vi "Match_Proc_STD Unit.vi"(10 "Cal STD 입력":string[][](array[string]), 11 "Condition Default":string[][](array[string])) -> (1 "Cal STD 출력":string[][](array[string]), 2 "Unit":string, 3 "Condition Default out":string[][](array[string]), 4 "STD ≥ DUT?":bool, 5 "x < 0?":bool)   [LabVIEW 2020]
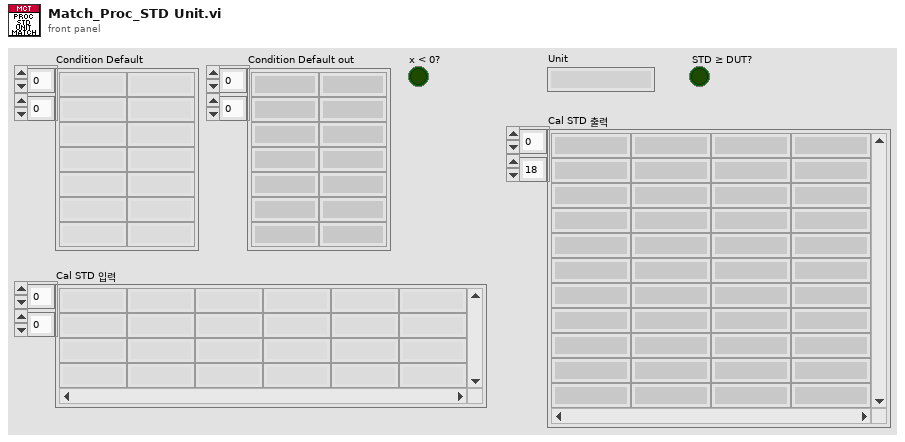
[diagram p1: front panel]
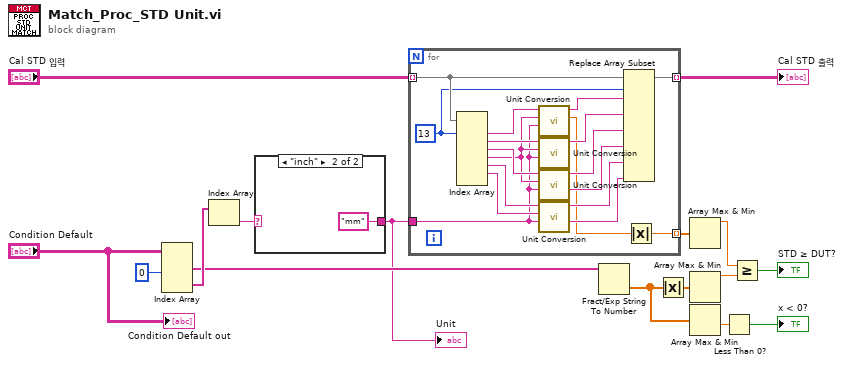
[diagram p0: block diagram]
diagram:
  n1 = Index Array(array="Condition Default", index (col) #1=0 ("비활성화된 인덱스 (열)")) -> (element #1=w15:string[], element #2=w16:string[])  [unwired: 3 in]
  n2 = Index Array(array=w16) -> (element=w6:string)  [unwired: 1 in]
  n3 = case shown="\"inch\"" w6 {
    selector: w6 -> [w17 _]
    tunnel: [w17 "mm"] -> w5
    frame Default {
    }
    frame "inch" {
    }
  }
  "Unit" <- w5
  n4 = for {
    tunnel: "Cal STD 입력" -> [w34] mode=indexing
    tunnel: w5 -> [w25]
    tunnel: [w30] -> w8 mode=indexing
    tunnel: [w19] -> w9 mode=indexing
    w33 = 13 ("인덱스 (행)")
    n5 = Index Array(array=w34, index #1=w33) -> (element #1=w36:string, element #2=w35:string, element #3=w29:string, element #4=w28:string, element #5=w27:string, element #6=w26:string)  [unwired: 6 in, 1 out]
    n6 = call "Unit Conversion.vi"("환산단위"=w25, "입력단위"=w28, "입력값"=w36) -> ("환산값 (DBL)"=w20:dbl, "환산값 (string)"=w32:string)  [unwired: 3 in, 4 out]
    n7 = call "Unit Conversion.vi"("환산단위"=w25, "입력단위"=w28, "입력값"=w35) -> ("환산값 (string)"=w31:string)  [unwired: 3 in, 5 out]
    n8 = call "Unit Conversion.vi"("환산단위"=w25, "입력단위"=w28, "입력값"=w29) -> ("환산단위"=w23:string, "환산값 (string)"=w24:string)  [unwired: 3 in, 4 out]
    n9 = call "Unit Conversion.vi"("환산단위"=w25, "입력단위"=w26, "입력값"=w27) -> ("환산단위"=w21:string, "환산값 (string)"=w22:string)  [unwired: 3 in, 4 out]
    n10 = Replace Array Subset(array=w34, new element #1=w32, index #1=w33, new element #2=w31, new element #3=w24, new element #4=w23, new element #5=w22, new element #6=w21) -> (w30:string[])  [unwired: 5 in]
    n11 = Absolute Value(x=w20) -> (abs(x)=w19:dbl)
  }
  "Cal STD 출력" <- w8
  n12 = Fract/Exp String To Number(string=w15) -> (number=w3:dbl[])  [unwired: 3 in, 1 out]
  n13 = Absolute Value(x=w3) -> (abs(x)=w12:dbl[])
  n14 = Array Max & Min(array=w9) -> (max value=w10:dbl)  [unwired: 3 out]
  n15 = Array Max & Min(array=w12) -> (max value=w11:dbl)  [unwired: 3 out]
  n16 = Array Max & Min(array=w3) -> (min value=w4:dbl)  [unwired: 3 out]
  n17 = Less Than 0?(x=w4) -> (x < 0?=→"x < 0?":bool)
  n18 = Greater Or Equal?(x=w10, y=w11) -> (x >= y?=→"STD ≥ DUT?":bool)
  "Condition Default out" <- "Condition Default"
